vi "Notebook.vi"() -> ()   [LabVIEW 2019, in "Notebook.lvlib"]
uses:
  Notebook.lvlib
  System.Windows.Forms
  Notebook Action Q Element.ctl
  Notebook Action List.ctl
  System.Drawing
  Text Colors.ctl
  Formatted Text.ctl
  Text Formatting.ctl
  Notebook Saved Global.vi
  Notebook Main VI Name.vi
  Rich Text Box.lvlib
  Variant to Data.lvlib
panel:
  in  "Notebook Content":refnum<k24>(container)
types:
  T1 = enum32{"Invalid", "Standard", "Closed", "Hidden", "Minimized", "Maximized"}
  T2 = typedef "Notebook.lvlib/Notebook Action Q Element.ctl" = cluster{"Action":T3, "Variant":variant}
  T3 = typedef "Notebook.lvlib/Notebook Action List.ctl" = enum16{"Idle", "Init", "Check Content Change", "User added content", "Program added text", "Program added Picture ", "Save Notebook", "Quit", "Open", "Close", "Update Window Title"}
  T4 = typedef "Rich Text Box.lvlib/Text Colors.ctl" = enum16{"Unchanged", "Black", "Blue", "Gray", "Green", "Red", "White"}
  T5 = typedef "Rich Text Box.lvlib/Formatted Text.ctl" = cluster{"Text":string, "Text Formatting":T6}
  T6 = typedef "Rich Text Box.lvlib/Text Formatting.ctl" = cluster{"Font":string, "Text Color":T4, "Text Background Color":T4, "Text Style":enum16{"Regular", "Bold", "Italic", "Underline", "Strikeout"}, "Font Size (Points)":dbl, "Text Alignment":i32}
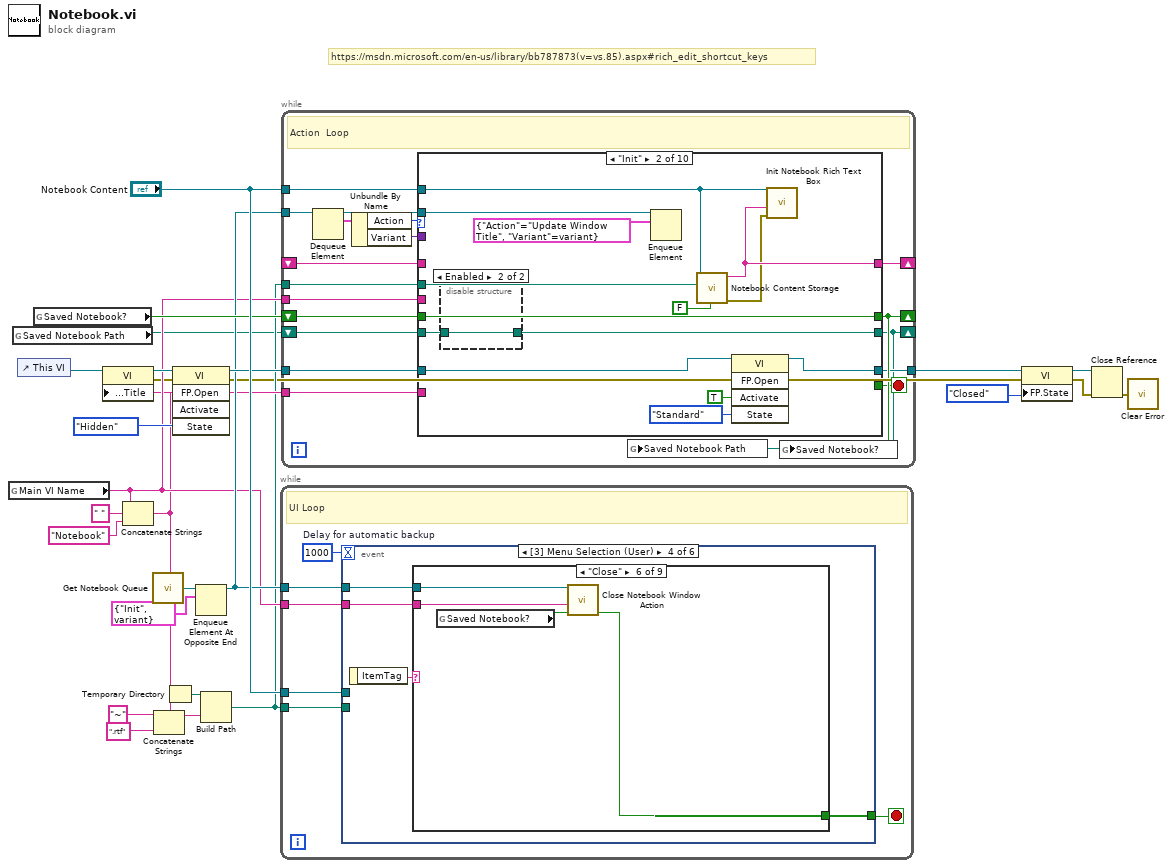
[diagram p0: block diagram]
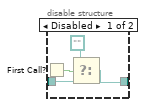
[diagram p3: hidden frame]
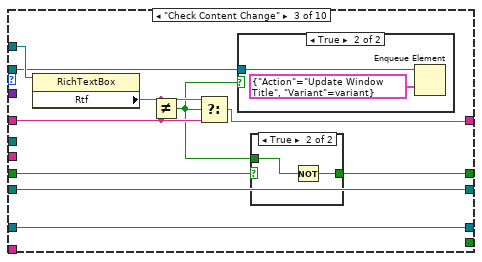
[diagram p4: hidden frame]
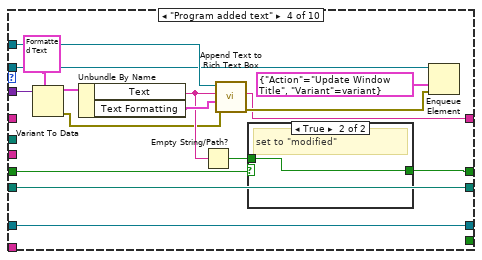
[diagram p7: hidden frame]
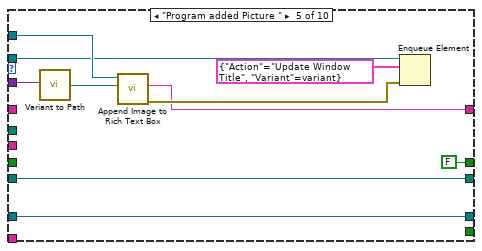
[diagram p9: hidden frame]
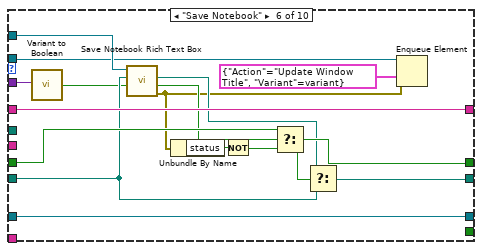
[diagram p10: hidden frame]
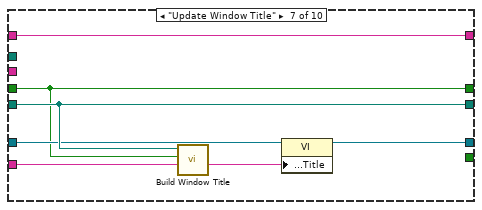
[diagram p11: hidden frame]
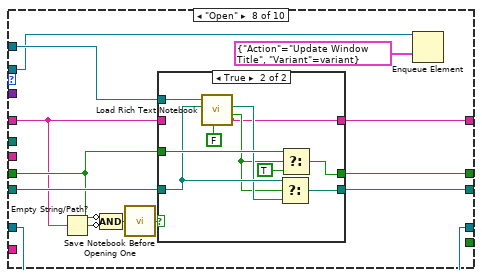
[diagram p12: hidden frame]
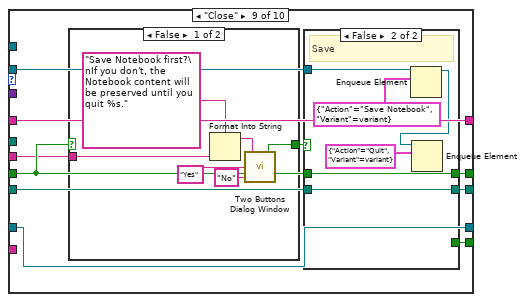
[diagram p14: hidden frame]
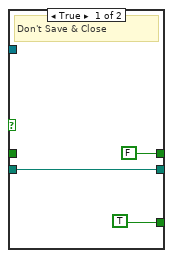
[diagram p15: hidden frame]
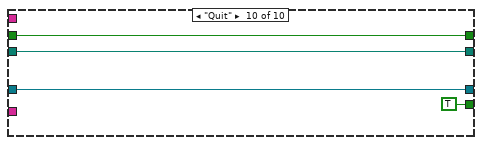
[diagram p17: hidden frame]
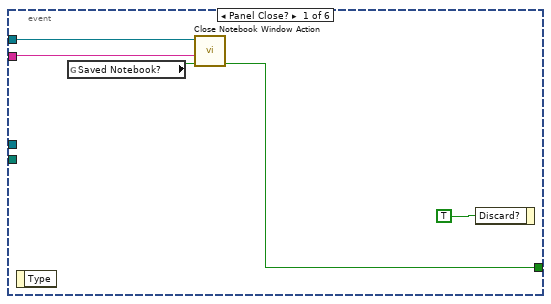
[diagram p18: hidden frame]
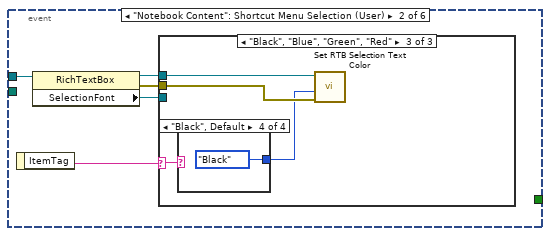
[diagram p19: hidden frame]
diagram:
  # "https://msdn.microsoft.com/en-us/library/bb787873(v=vs.85).aspx#rich_edit_shortcut_keys"
  n1 = global read "Notebook Main VI Name.vi" "Main VI Name"() -> (w11:string)
  n2 = global read "Notebook Saved Global.vi" "Saved Notebook Path"() -> (w5:path)
  n3 = control-ref of="This VI"() -> (w21:refnum<vi>)
  n4 = global read "Notebook Saved Global.vi" "Saved Notebook?"() -> (w18:bool)
  n5 = Concatenate Strings(w11, " " ("string"), "Notebook" ("string")) -> (w9:string)
  n6 = property class="VI"(reference=w21, "Front Panel.Title"=w9) -> (reference out=w15:refnum<vi>, error out=w4:errorcluster)  [unwired: 1 in]
  n7 = call "Get Notebook Queue.vi"() -> ("Notebook Queue"=w17:refnum<queue>)  [unwired: 9 in]
  n8 = Concatenate Strings("~" ("string"), w9, ".rtf" ("format string")) -> (w7:string)
  n9 = Temporary Directory() -> (w22:path)
  n10 = invoke class="VI" method="FP.Open"(reference=w15, error in=w4, "State"=T1."Hidden") -> (reference out=w20:refnum<vi>, error out=w3:errorcluster)  [unwired: 2 in, 3 out]
  n11 = Enqueue Element At Opposite End(queue=w17, element=T2 {"Action"=enum."Init", "Variant"=variant}) -> (queue out=w16:refnum<queue>)  [unwired: 2 in, 2 out]
  n12 = Build Path(base path=w22, name or relative path=w7) -> (appended path=w6:path)
  n13 = while {
    tunnel: w16 -> [w31]
    tunnel: "Notebook Content" -> [w29]
    tunnel: w11 -> [w27]
    tunnel: w6 -> [w28]
    stop <- w32 stop-if-true
    w30 = 1000  # Delay for automatic backup
    # "UI Loop"
    n14 = event shown="[3] Menu Selection (User)" {
      selector: _ -> [_ _ _ _ _ _]
      dyn-events: _ -> [_ _ _ _ _ _]
      timeout: w30 -> [_ _ _ _ _ _]
      tunnel: [w36 _ _ w72 w100 _] -> w32
      tunnel: w31 -> [w37 _ w70 w73 w101 _]
      tunnel: w29 -> [_ w41 w68 _ _ w114]
      tunnel: w28 -> [_ _ w67 _ _ _]
      tunnel: w27 -> [w33 _ _ w71 w99 _]
      event Panel Close? {
        n15 = event-data() -> ()  [unwired: 1 in, 1 out]
        n16 = global read "Notebook Saved Global.vi" "Saved Notebook?"() -> (w34:bool)
        n17 = call "Close Notebook Window Action.vi"("Notebook Saved?"=w34, "Main VI Name"=w33, "Notebook Queue"=w37) -> ("Quit?"=w36:bool)  [unwired: 8 in]
        n18 = event-data("Discard?"=TRUE) -> ()  [unwired: 1 in, 1 out]
      }
      event "Notebook Content": Shortcut Menu Selection (User) {
        n19 = event-data() -> ("ItemTag"=w42:string)  [unwired: 1 in]
        n20 = property class="RichTextBox"(reference=w41) -> (reference out=w38:refnum<k24>, error out=w39:errorcluster, "SelectionFont"=w40:refnum<k24>)  [unwired: 1 in]
        n21 = case shown="\"Black\", \"Blue\", \"Green\", \"Red\"" w42 {
          selector: w42 -> [_ w48 w59]
          tunnel: w40 -> [_ w52 _]
          tunnel: w39 -> [_ w47 w60]
          tunnel: w38 -> [_ w44 w61]
          frame "", Default {
          }
          frame "Bold", "Italic", "Regular", "Strikeout", "Underline" {
            n22 = property class="Font"(reference=w52, error in=w47) -> (error out=w46:errorcluster, "Name"=w51:string, "SizeInPoints"=w50:sgl)  [unwired: 1 out]
            n23 = case shown="\"Bold\"" w48 {
              tunnel: [w53 w54 w55 w56 w57] -> w49
              frame "Regular", Default {
                w53 = 0 items=["Regular"=0, "Bold"=1, "Italic"=2, "Underline"=4, "Strikeout"=8] ("style")
              }
              frame "Bold" {
                w54 = 1 items=["Regular"=0, "Bold"=1, "Italic"=2, "Underline"=4, "Strikeout"=8] ("style")
              }
              frame "Italic" {
                w55 = 2 items=["Regular"=0, "Bold"=1, "Italic"=2, "Underline"=4, "Strikeout"=8] ("style")
              }
              frame "Underline" {
                w56 = 4 items=["Regular"=0, "Bold"=1, "Italic"=2, "Underline"=4, "Strikeout"=8] ("style")
              }
              frame "Strikeout" {
                w57 = 8 items=["Regular"=0, "Bold"=1, "Italic"=2, "Underline"=4, "Strikeout"=8] ("style")
              }
            }
            n24 = constructor class="Font"(error in=w46, "familyName"=w51, "emSize"=w50, "unit"=w49) -> (reference out=w43:refnum<k24>, error out=w45:errorcluster)  [unwired: 2 in, 4 out]
            n25 = property class="RichTextBox"(reference=w44, error in=w45, "SelectionFont"=w43) -> ()  [unwired: 2 out]
          }
          frame "Black", "Blue", "Green", "Red" {
            n26 = case shown="\"Black\", Default" w59 {
              tunnel: [Text_Colors."Blue" ("Text Color") Text_Colors."Green" ("Text Color") Text_Colors."Red" ("Text Color") Text_Colors."Black" ("Text Color")] -> w58
              frame "Blue" {
              }
              frame "Green" {
              }
              frame "Red" {
              }
              frame "Black", Default {
              }
            }
            n27 = call "Set RTB Selection Text Color.vi"("Error In"=w60, "Text Color"=w58, ".NET RTB Refnum in"=w61) -> ()  [unwired: 7 in, 2 out]
          }
        }
      }
      event Timeout {
        n28 = event-data() -> ()  [unwired: 1 in, 1 out]
        n29 = call "Notebook Content Storage.vi"("Save(T)/Load(F)"=TRUE, "path"=w67, ".NET Refnum in"=w68) -> ()  [unwired: 7 in, 2 out]
        n30 = Enqueue Element(queue=w70, element=T2 {"Action"=enum."Check Content Change", "Variant"=variant}) -> ()  [unwired: 2 in, 3 out]
      }
      event Menu Selection (User) {
        n31 = event-data() -> ("ItemTag"=w74:string)  [unwired: 1 in]
        n32 = case shown="\"Close\"" w74 {
          tunnel: w73 -> [_ _ w76 w80 w84 w88 _ w98 _]
          tunnel: [_ _ _ _ _ w87 _ _ _] -> w72
          tunnel: w71 -> [_ _ _ _ _ w85 _ _ _]
          frame "", Default {
          }
          frame "---------File----------" {
          }
          frame "Open" {
            n33 = Enqueue Element(queue=w76, element=T2 {"Action"=enum."Open", "Variant"=variant}) -> ()  [unwired: 2 in, 3 out]
          }
          frame "Save" {
            w77 = FALSE  # No dialog
            n34 = Bundle By Name(cluster=T2 {"Action"=enum."Save Notebook", "Variant"=variant} ("element"), "Variant"=w77) -> (w78:T2)
            n35 = Enqueue Element(queue=w80, element=w78) -> ()  [unwired: 2 in, 3 out]
          }
          frame "Save As" {
            w81 = TRUE  # Dialog
            n36 = Bundle By Name(cluster=T2 {"Action"=enum."Save Notebook", "Variant"=variant} ("element"), "Variant"=w81) -> (w82:T2)
            n37 = Enqueue Element(queue=w84, element=w82) -> ()  [unwired: 2 in, 3 out]
          }
          frame "Close" {
            n38 = global read "Notebook Saved Global.vi" "Saved Notebook?"() -> (w86:bool)
            n39 = call "Close Notebook Window Action.vi"("Notebook Saved?"=w86, "Main VI Name"=w85, "Notebook Queue"=w88) -> ("Quit?"=w87:bool)  [unwired: 8 in]
          }
          frame "----------Edit----------" {
          }
          frame "Paste Current Date & Time" {
            n40 = call "Current Date & Time String.vi"() -> ("time string"=w89:string, "date string"=w90:string)  [unwired: 9 in, 1 out]
            n41 = Format Into String(format string="Current Date & Time: %s, %s" ("initial string"), w90, w89) -> (resulting string=w93:string)  [unwired: 2 in, 1 out]
            n42 = call "Message Style.vi"() -> ("Message Formatting"=w92:T6)
            n43 = Bundle By Name(cluster=T5 {"Text"="", "Text Formatting"={"Font"="Default", "Text Color"=enum."Unchanged", "Text Background Color"=enum."Unchanged", "Text Style"=enum."Regular", "Font Size (Points)"=-1.0, "Text Alignment"=0}} ("Formatted Text"), "Text"=w93, "Text Formatting"=w92) -> (w94:T5)
            n44 = Bundle By Name(cluster=T2 {"Action"=enum."Program added text", "Variant"=variant} ("element"), "Variant"=w94) -> (w96:T2)
            n45 = Enqueue Element(queue=w98, element=w96) -> ()  [unwired: 2 in, 3 out]
          }
          frame "Find..." {
          }
        }
      }
      event "Notebook Content": Shortcut Menu Selection (App) {
        n46 = event-data() -> ("ItemTag"=w102:string)  [unwired: 1 in, 1 out]
        n47 = case shown="\"Paste Current Date & Time\"" w102 {
          tunnel: w101 -> [_ w113]
          tunnel: [_ FALSE ("Quit?")] -> w100
          tunnel: w99 -> [_ _]
          frame "", Default {
          }
          frame "Paste Current Date & Time" {
            n48 = call "Current Date & Time String.vi"() -> ("time string"=w105:string, "date string"=w104:string)  [unwired: 9 in, 1 out]
            n49 = Format Into String(format string="Current Date & Time: %s, %s" ("initial string"), w104, w105) -> (resulting string=w108:string)  [unwired: 2 in, 1 out]
            n50 = call "Message Style.vi"() -> ("Message Formatting"=w107:T6)
            n51 = Bundle By Name(cluster=T5 {"Text"="", "Text Formatting"={"Font"="Default", "Text Color"=enum."Unchanged", "Text Background Color"=enum."Unchanged", "Text Style"=enum."Regular", "Font Size (Points)"=-1.0, "Text Alignment"=0}} ("Formatted Text"), "Text"=w108, "Text Formatting"=w107) -> (w109:T5)
            n52 = Bundle By Name(cluster=T2 {"Action"=enum."Program added text", "Variant"=variant} ("element"), "Variant"=w109) -> (w111:T2)
            n53 = Enqueue Element(queue=w113, element=w111) -> ()  [unwired: 2 in, 3 out]
          }
        }
      }
      event Panel Resize {
        n54 = event-data() -> ()  [unwired: 1 in, 1 out]
        n55 = disable-structure shown="Enabled" {
          disable-tunnel: w114 -> [_ w116]
          frame Disabled {
            w115 = inf
          }
          frame Enabled {
            n56 = invoke class="RichTextBox" method="ScrollToCaret"(reference=w116) -> ()  [unwired: 2 in, 3 out]
          }
        }
      }
    }
  }
  n57 = while {
    tunnel: w16 -> [w134]
    shift-right: [w127] -> _
    shift-left: w18 -> [w131]
    shift-right: [w117] -> _
    shift-left: w5 -> [w130]
    tunnel: w20 -> [w124]
    tunnel: [w122] -> w26
    tunnel: "Notebook Content" -> [w126]
    tunnel: w11 -> [w123]
    tunnel: w9 -> [w121]
    shift-right: [w120] -> _
    shift-left: _ -> [w119]
    tunnel: w6 -> [w118]
    stop <- w125 stop-if-true
    # "Action  Loop"
    n58 = Dequeue Element(queue=w134) -> (queue out=w129:refnum<queue>, element=w133:T2)  [unwired: 2 in, 2 out]
    n59 = Unbundle By Name(w133) -> ("Action"=w132:T3, "Variant"=w128:variant)
    n60 = case shown="\"Init\"" w132 {
      tunnel: w131 -> [w138 w139 w160 w175 _ w212 w219 w233 w254 w279]
      tunnel: [w138 w139 w159 w174 FALSE ("Saved?") w207 w219 w234 w258 w279] -> w127
      tunnel: w130 -> [w137 w149 w167 w188 w200 w209 w223 w236 w256 w278]
      tunnel: [w137 w148 w167 w188 w200 w210 w223 w235 w255 w278] -> w117
      tunnel: w129 -> [_ w141 w161 w177 w193 w206 _ w226 w257 _]
      tunnel: w128 -> [_ _ _ w186 w198 w204 _ _ _ _]
      tunnel: w126 -> [_ w143 w165 w187 w199 w216 _ w229 _ _]
      tunnel: [_ _ _ _ _ _ _ _ w253 TRUE] -> w125
      tunnel: w124 -> [w136 w152 w166 w180 w195 w213 w221 w228 w251 w276]
      tunnel: w123 -> [_ _ _ _ _ _ _ _ w252 _]
      tunnel: [w136 w147 w166 w180 w195 w213 w220 w228 w251 w276] -> w122
      tunnel: w121 -> [_ _ _ _ _ _ w218 _ _ _]
      tunnel: [w135 w146 w162 w176 w191 w211 w217 w225 w250 _] -> w120
      tunnel: w119 -> [w135 _ w163 _ _ w211 w217 w224 w250 _]
      tunnel: w118 -> [_ w144 _ _ _ _ _ _ _ _]
      frame "Idle", Default {
      }
      frame "Init" {
        n61 = disable-structure shown="Enabled" {
          disable-tunnel: w149 -> [w156 w157]
          disable-tunnel: [w155 w157] -> w148
          frame Disabled {
            n62 = First Call?() -> (First Call?: T/F=w153:bool)
            n63 = Select(t=path "", s=w153, f=w156) -> (s? t:f=w155:path)
          }
          frame Enabled {
          }
        }
        n64 = Enqueue Element(queue=w141, element=T2 {"Action"=enum."Update Window Title", "Variant"=variant}) -> ()  [unwired: 2 in, 3 out]
        n65 = call "Notebook Content Storage.vi"("Save(T)/Load(F)"=FALSE ("Set(T)/Get(F)"), "path"=w144, ".NET Refnum in"=w143) -> ("Error Out"=w142:errorcluster, "RTF content"=w146:string)  [unwired: 7 in]
        n66 = invoke class="VI" method="FP.Open"(reference=w152, "Activate"=TRUE ("Activate?"), "State"=T1."Standard") -> (reference out=w147:refnum<vi>)  [unwired: 2 in, 4 out]
        n67 = call "Init Notebook Rich Text Box.vi"("Error In"=w142, "Notebook Content"=w146, ".NET Refnum in"=w143) -> ()  [unwired: 8 in, 1 out]
      }
      frame "Check Content Change" {
        n68 = property class="RichTextBox"(reference=w165) -> ("Rtf"=w164:string)  [unwired: 1 in, 2 out]
        n69 = Not Equal?(x=w164, y=w163) -> (x != y?=w158:bool)
        n70 = Select(t=w164, s=w158, f=w163) -> (s? t:f=w162:string)
        n71 = case shown="True" w158 {
          tunnel: w161 -> [_ w172]
          frame False {
          }
          frame True {
            n72 = Enqueue Element(queue=w172, element=T2 {"Action"=enum."Update Window Title", "Variant"=variant}) -> ()  [unwired: 2 in, 3 out]
          }
        }
        n73 = case shown="True" w160 {
          selector: w160 -> [w168 _]
          tunnel: [w168 w169] -> w159
          tunnel: w158 -> [_ w170]
          frame False {
          }
          frame True {
            n74 = Not(x=w170) -> (.not. x?=w169:bool)
          }
        }
      }
      frame "Program added text" {
        n75 = Variant To Data(type=T5 {"Text"="", "Text Formatting"={"Font"="Default", "Text Color"=enum."Unchanged", "Text Background Color"=enum."Unchanged", "Text Style"=enum."Regular", "Font Size (Points)"=-1.0, "Text Alignment"=0}} ("Formatted Text"), Variant=w186) -> (data=w184:T5, error out=w181:errorcluster)  [unwired: 1 in]
        n76 = Unbundle By Name(w184) -> ("Text"=w182:string, "Text Formatting"=w183:T6)
        n77 = Empty String/Path?(string/path=w182) -> (empty?=w173:bool)
        n78 = call "Append Text to Rich Text Box.vi"("error in (no error)"=w181, "Text Formatting"=w183, "String"=w182, ".NET Refnum in"=w187) -> ("Error Out"=w178:errorcluster, "Rtf Content"=w176:string)  [unwired: 6 in]
        n79 = case shown="True" w175 {
          selector: w175 -> [w189 _]
          tunnel: [w189 w190] -> w174
          tunnel: w173 -> [_ w190]
          frame False {
            # "remains \"modified\""
          }
          frame True {
            # "set to \"modified\""
          }
        }
        n80 = Enqueue Element(queue=w177, element=T2 {"Action"=enum."Update Window Title", "Variant"=variant}, error in (no error)=w178) -> ()  [unwired: 1 in, 3 out]
      }
      frame "Program added Picture " {
        n81 = call "Variant to Path.vi"("Variant"=w198) -> ("Path"=w197:path)  [unwired: 8 in]
        n82 = call "Append Image to Rich Text Box.vi"("Image File Path"=w197, ".NET Refnum in"=w199) -> ("error out"=w192:errorcluster, "Rtf Content"=w191:string)  [unwired: 8 in]
        n83 = Enqueue Element(queue=w193, element=T2 {"Action"=enum."Update Window Title", "Variant"=variant}, error in (no error)=w192) -> ()  [unwired: 1 in, 3 out]
      }
      frame "Save Notebook" {
        n84 = call "Variant to Boolean.vi"("Variant"=w204) -> ("Value"=w203:bool)  [unwired: 8 in]
        n85 = call "Save Notebook Rich Text Box.vi"("Dialog (F)"=w203, "File Path Control"=w209, ".NET Refnum in"=w216) -> ("Error Out"=w201:errorcluster, "cancelled"=w208:bool, "File Path out"=w202:path)  [unwired: 6 in]
        n86 = Unbundle By Name(w201) -> ("status"=w215:bool)
        n87 = Not(x=w215) -> (.not. x?=w214:bool)
        n88 = Select(t=w212, s=w208, f=w214) -> (s? t:f=w207:bool)
        n89 = Select(t=w202, s=w207, f=w209) -> (s? t:f=w210:path)
        n90 = Enqueue Element(queue=w206, element=T2 {"Action"=enum."Update Window Title", "Variant"=variant}, error in (no error)=w201) -> ()  [unwired: 1 in, 3 out]
      }
      frame "Update Window Title" {
        n91 = call "Build Window Title.vi"("Root Window Title"=w218, "Saved Notebook?"=w219, "File Path in"=w223) -> ("Modified Window Title"=w222:string)  [unwired: 8 in]
        n92 = property class="VI"(reference=w221, "Front Panel.Title"=w222) -> (reference out=w220:refnum<vi>)  [unwired: 1 in, 1 out]
      }
      frame "Open" {
        n93 = Empty String/Path?(string/path=w224) -> (empty?=w230:bool)
        n94 = Compound Arithmetic op=AND(invert w233, invert w230) -> (w232:bool)
        n95 = call "Save Notebook Before Opening One.vi"("Not saved?"=w232) -> ("Save?"=w231:bool)  [unwired: 8 in]
        n96 = case shown="True" w231 {
          tunnel: w236 -> [w238 w247]
          tunnel: [w238 w246] -> w235
          tunnel: [w239 w249] -> w234
          tunnel: w233 -> [w239 w248]
          tunnel: w229 -> [_ w245]
          tunnel: [w237 w241] -> w225
          tunnel: w224 -> [w237 _]
          frame False {
          }
          frame True {
            n97 = call "Load Rich Text Notebook.vi"("Backup?"=FALSE, "File Path Control"=w247, ".NET Refnum in"=w245) -> ("cancelled"=w243:bool, "File Path out"=w244:path, "RTF content"=w241:string)  [unwired: 4 in, 2 out]
            n98 = Select(t=w247, s=w243, f=w244) -> (s? t:f=w246:path)
            n99 = Select(t=w248, s=w243, f=TRUE) -> (s? t:f=w249:bool)
          }
        }
        n100 = Enqueue Element(queue=w226, element=T2 {"Action"=enum."Update Window Title", "Variant"=variant}) -> ()  [unwired: 2 in, 3 out]
      }
      frame "Close" {
        n101 = case shown="False" w254 {
          selector: w254 -> [_ w275]
          tunnel: [w273 w275] -> w259
          tunnel: w252 -> [w269 _]
          frame False {
            n102 = Format Into String(format string="Save Notebook first?\nIf you don't, the Notebook content will be preserved until you quit %s." ("message"), w269) -> (resulting string=w271:string)  [unwired: 2 in, 1 out]
            n103 = call "Two Buttons Dialog Window.vi"("Cancel Button Text"="No" ("F button name (\"Cancel\")"), "OK Button Text"="Yes" ("T button name (\"OK\")"), "Message"=w271) -> ("OK?"=w273:bool)
          }
          frame True {
          }
        }
        n104 = case shown="False" w259 {
          tunnel: w254 -> [_ w266]
          tunnel: [FALSE ("Saved?") w266] -> w258
          tunnel: w257 -> [_ w268]
          tunnel: w256 -> [w261 w265]
          tunnel: [w261 w265] -> w255
          tunnel: [TRUE _] -> w253
          frame True {
            # "Don't Save & Close"
          }
          frame False {
            # "Save"
            n105 = Enqueue Element(queue=w268, element=T2 {"Action"=enum."Save Notebook", "Variant"=variant}) -> (queue out=w263:refnum<queue>)  [unwired: 2 in, 2 out]
            n106 = Enqueue Element(queue=w263, element=T2 {"Action"=enum."Quit", "Variant"=variant}) -> ()  [unwired: 2 in, 3 out]
          }
        }
      }
      frame "Quit" {
      }
    }
    n107 = global write "Notebook Saved Global.vi" "Saved Notebook Path"(w117) -> ()
    n108 = global write "Notebook Saved Global.vi" "Saved Notebook?"(w127) -> ()
  }
  n109 = property class="VI"(reference=w26, error in=w3, "FP.State"=T1."Closed" ("Front Panel Window:State")) -> (reference out=w24:refnum<vi>, error out=w2:errorcluster)
  n110 = Close Reference(reference=w24, error in (no error)=w2) -> (error out=w1:errorcluster)
  n111 = call "Clear Error.vi"("Error In"=w1) -> ()  [unwired: 8 in, 1 out]
